vi "A cross diagonal.vi"(10 "diagonal":dbl[](array[numeric]), 11 "A":T1) -> (3 "Axdiagonal":T1)   [LabVIEW 2020, in "NI_Gmath.lvlib"]
uses:
  NI_Gmath.lvlib
  RealMatrix.ctl
  NI_Matrix.lvlib
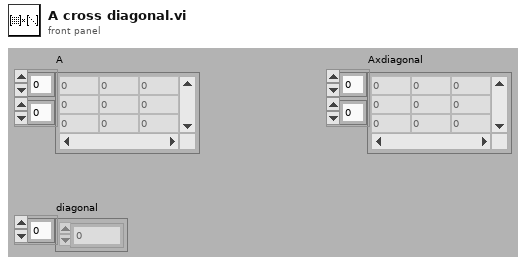
[diagram p1: front panel]
types:
  T1 = typedef "NI_Matrix.lvlib/RealMatrix.ctl" = dbl[][]
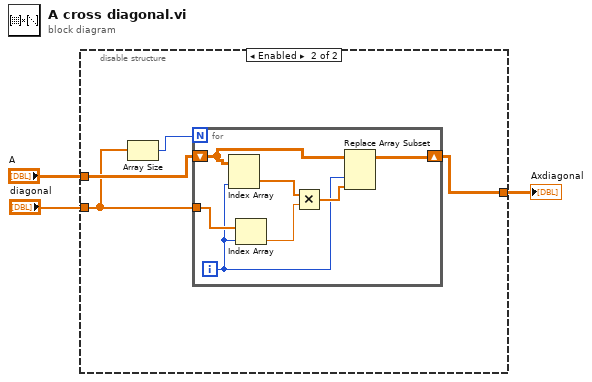
[diagram p0: block diagram]
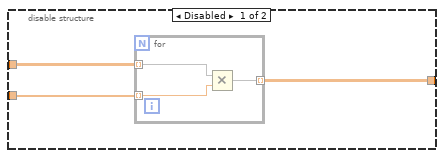
[diagram p2: hidden frame]
diagram:
  n1 = disable-structure shown="Enabled" {
    disable-tunnel: "A" -> [w6 w13]
    disable-tunnel: "diagonal" -> [w5 w11]
    disable-tunnel: [w4 w12] -> w1
    frame Disabled {
      n2 = for {
        tunnel: w6 -> [w9] mode=indexing
        tunnel: w5 -> [w8] mode=indexing
        tunnel: [w7] -> w4 mode=indexing
        n3 = Multiply(x=w9, y=w8) -> (x*y=w7:dbl[])
      }
    }
    frame Enabled {
      n4 = Array Size(array=w11) -> (size(s)=w10:i32)
      n5 = for {
        N: w10 -> [_]
        tunnel: w11 -> [w16]
        shift-right: [w17] -> w12
        shift-left: w13 -> [w20]
        i -> [w14]
        n6 = Index Array(array=w20, index (col)=w14) -> (element=w19:dbl[])  [unwired: 1 in]
        n7 = Index Array(array=w16, index=w14) -> (element=w15:dbl)
        n8 = Multiply ("Multiply.vi")(x=w19, y=w15) -> (x*y=w18:dbl[])
        n9 = Replace Array Subset(array=w20, new element=w18, index (col)=w14) -> (w17:T1)  [unwired: 1 in]
      }
    }
  }
  "Axdiagonal" <- w1
